vi "TC_N_VtoC.vi"(11 "Thermocouple Voltage":dbl caption="热电偶电压" format="%0.6f") -> (3 "T(c)":dbl format="%#_16f")   [LabVIEW 2012]
doc: "功能：\n\nE型热电偶电压转换为摄氏度。\n\ncsxcs_366创建。"
uses:
  <vilib>/Analysis/polynomials.llb/Scalar Polynomial Evaluation (DBL).vi
  <vilib>/Analysis/NI_AALPro.lvlib
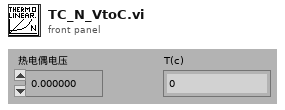
[diagram p1: front panel]
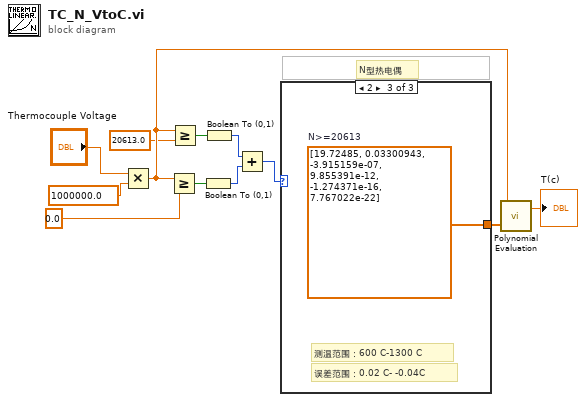
[diagram p0: block diagram]
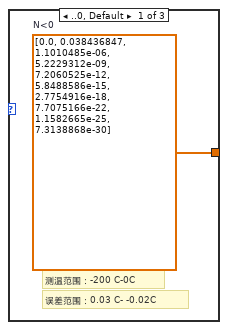
[diagram p2: hidden frame]
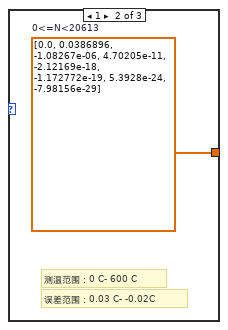
[diagram p3: hidden frame]
diagram:
  # "N型热电偶"
  n1 = Multiply(x="Thermocouple Voltage", y=1000000.0) -> (x*y=w8:dbl)
  n2 = Greater Or Equal?(x=w8, y=0.0) -> (x >= y?=w5:bool)
  n3 = Greater Or Equal?(x=w8, y=20613.0) -> (x >= y?=w6:bool)
  n4 = Boolean To (0,1)(Boolean=w5) -> (0, 1=w4:i16)
  n5 = Boolean To (0,1)(Boolean=w6) -> (0, 1=w3:i16)
  n6 = Add(x=w3, y=w4) -> (x+y=w2:i16)
  n7 = case shown="2" w2 {
    tunnel: [w13 w14 w15] -> w1
    frame ..0, Default {
      w13 = dbl[] [0.0, 0.038436847, 1.1010485e-06, 5.2229312e-09, 7.2060525e-12, 5.8488586e-15, 2.7754916e-18, 7.7075166e-22, 1.1582665e-25, 7.3138868e-30]  # N<0
      # "误差范围：0.03 C- -0.02C"
      # "测温范围：-200 C-0C"
    }
    frame 1 {
      w14 = dbl[] [0.0, 0.0386896, -1.08267e-06, 4.70205e-11, -2.12169e-18, -1.172772e-19, 5.3928e-24, -7.98156e-29]  # 0<=N<20613
      # "误差范围：0.03 C- -0.02C"
      # "测温范围：0 C- 600 C"
    }
    frame 2 {
      w15 = dbl[] [19.72485, 0.03300943, -3.915159e-07, 9.855391e-12, -1.274371e-16, 7.767022e-22]  # N>=20613
      # "误差范围：0.02 C- -0.04C"
      # "测温范围：600 C-1300 C"
    }
  }
  n8 = call-poly <vilib>:"Polynomial Evaluation.vi"("P(x)"=w1, "a"=w8) -> ("P(a)"=→"T(c)":dbl)  [unwired: 1 out]
